vi "fetch frame gige.vi"() -> ()   [LabVIEW 2015]
uses:
  <vilib>/Utility/miscctls.llb/LV3DPointTypeDef.ctl
  <vilib>/Utility/miscctls.llb/LVRGBAColorTypeDef.ctl
  <vilib>/picture/3D Picture Control/Object/Create Object (name).vi
  <userlib>/Mv3dRgbd/Mv3dRgbd.lvlib
  <vilib>/picture/3D Picture Control/NI_3D Picture Control.lvlib
  <userlib>/Mv3dRgbdEx/Mv3dRgbdEx.lvlib
panel:
  in  "value 3":sgl[](array[numeric])
  out "size 5":i32
  out "address 4":i64
  in  "handle":u32
  out "pstU3DeviceInfo out":T1
  out "MV3D_RGBD_GigEDEVICE_INFO out 3":T2(array[cluster])
  out "function return":i32
  out "get list return":i32
  out "pDeviceCount out 2":u32
  out "value 2":u32
  out "open gige function":i32
  out "pstGigeDeviceInfo out 2":T3
  out "MV3D_RGBD_GigEDEVICE_INFO out 2":T4(array[cluster])
  out "get list return 2":i32
  out "pDeviceCount out 3":u32
  out "size 3":i32
  out "address 3":i64
  out "pYuvImgge out":T5
  out "yuv422torgb return":i32
  out "address 2":i64
  out "size 4":i32
  out "address 5":i64
  in  "value":u32
  in  "?":enum32{"RGBD", "点云"}(tab)
  out "RGB":picture
  out "Depth":i16[][](graph)
  out "?":refnum<vi>(3d-picture)
  out "depthtocloud return":i32
  out "handle out 2":u32
  out "pstDepthImage out":T5
  out "fetchframe handle out":u32
  out "fetchframe function":i32
  in  "?":bool
  out "close handle out":u32
  out "close function":i32
  out "start handle out":u32
  out "stop handle out":u32
  out "init function":i32
  out "release function":i32
  out "stop function":i32
  out "start function":i32
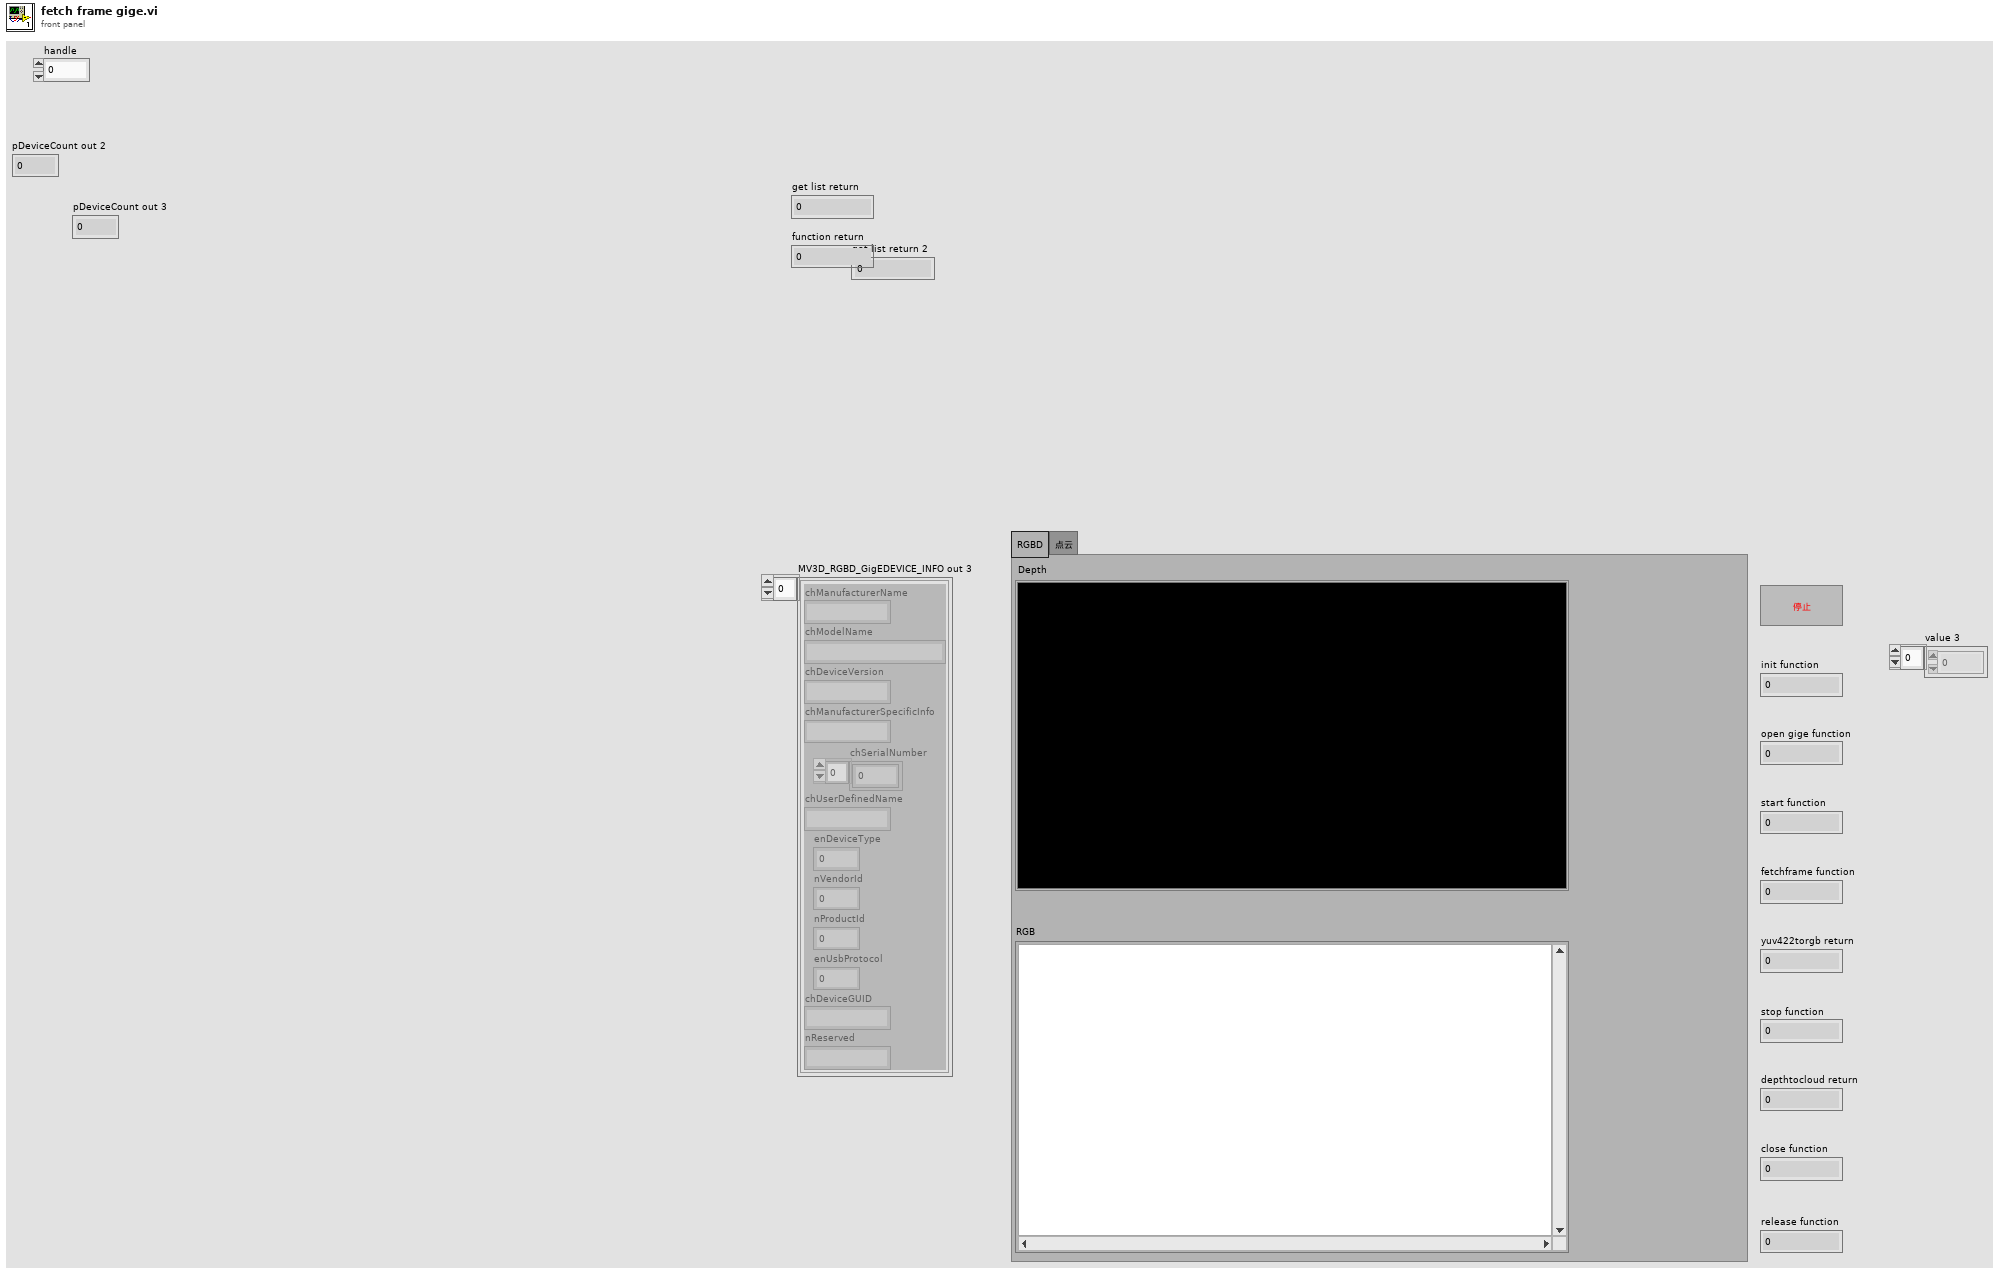
[diagram p1: front panel]
types:
  T1 = cluster{"chManufacturerName[0]":i8, "chManufacturerName[1]":i8, "chManufacturerName[2]":i8, "chManufacturerName[3]":i8, "chManufacturerName[4]":i8, "chManufacturerName[5]":i8, "chManufacturerName[6]":i8, "chManufacturerName[7]":i8, "chManufacturerName[8]":i8, "chManufacturerName[9]":i8, "chManufacturerName[10]":i8, "chManufacturerName[11]":i8, "chManufacturerName[12]":i8, "chManufacturerName[13]":i8, "chManufacturerName[14]":i8, "chManufacturerName[15]":i8, "chManufacturerName[16]":i8, "chManufacturerName[17]":i8, "chManufacturerName[18]":i8, "chManufacturerName[19]":i8, "chManufacturerName[20]":i8, "chManufacturerName[21]":i8, "chManufacturerName[22]":i8, "chManufacturerName[23]":i8, "chManufacturerName[24]":i8, "chManufacturerName[25]":i8, "chManufacturerName[26]":i8, "chManufacturerName[27]":i8, "chManufacturerName[28]":i8, "chManufacturerName[29]":i8, "chManufacturerName[30]":i8, "chManufacturerName[31]":i8, "chModelName[0]":i8, "chModelName[1]":i8, "chModelName[2]":i8, "chModelName[3]":i8, "chModelName[4]":i8, "chModelName[5]":i8, "chModelName[6]":i8, "chModelName[7]":i8, "chModelName[8]":i8, "chModelName[9]":i8, "chModelName[10]":i8, "chModelName[11]":i8, "chModelName[12]":i8, "chModelName[13]":i8, "chModelName[14]":i8, "chModelName[15]":i8, "chModelName[16]":i8, "chModelName[17]":i8, "chModelName[18]":i8, "chModelName[19]":i8, "chModelName[20]":i8, "chModelName[21]":i8, "chModelName[22]":i8, "chModelName[23]":i8, "chModelName[24]":i8, "chModelName[25]":i8, "chModelName[26]":i8, "chModelName[27]":i8, "chModelName[28]":i8, "chModelName[29]":i8, "chModelName[30]":i8, "chModelName[31]":i8, "chDeviceVersion[0]":i8, "chDeviceVersion[1]":i8, "chDeviceVersion[2]":i8, "chDeviceVersion[3]":i8, "chDeviceVersion[4]":i8, "chDeviceVersion[5]":i8, "chDeviceVersion[6]":i8, "chDeviceVersion[7]":i8, "chDeviceVersion[8]":i8, "chDeviceVersion[9]":i8, "chDeviceVersion[10]":i8, "chDeviceVersion[11]":i8, "chDeviceVersion[12]":i8, "chDeviceVersion[13]":i8, "chDeviceVersion[14]":i8, "chDeviceVersion[15]":i8, "chDeviceVersion[16]":i8, "chDeviceVersion[17]":i8, "chDeviceVersion[18]":i8, "chDeviceVersion[19]":i8, "chDeviceVersion[20]":i8, "chDeviceVersion[21]":i8, "chDeviceVersion[22]":i8, "chDeviceVersion[23]":i8, "chDeviceVersion[24]":i8, "chDeviceVersion[25]":i8, "chDeviceVersion[26]":i8, "chDeviceVersion[27]":i8, "chDeviceVersion[28]":i8, "chDeviceVersion[29]":i8, "chDeviceVersion[30]":i8, "chDeviceVersion[31]":i8, "chManufacturerSpecificInfo[0]":i8, "chManufacturerSpecificInfo[1]":i8, "chManufacturerSpecificInfo[2]":i8, "chManufacturerSpecificInfo[3]":i8, "chManufacturerSpecificInfo[4]":i8, "chManufacturerSpecificInfo[5]":i8, "chManufacturerSpecificInfo[6]":i8, "chManufacturerSpecificInfo[7]":i8, "chManufacturerSpecificInfo[8]":i8, "chManufacturerSpecificInfo[9]":i8, "chManufacturerSpecificInfo[10]":i8, "chManufacturerSpecificInfo[11]":i8, "chManufacturerSpecificInfo[12]":i8, "chManufacturerSpecificInfo[13]":i8, "chManufacturerSpecificInfo[14]":i8, "chManufacturerSpecificInfo[15]":i8, "chManufacturerSpecificInfo[16]":i8, "chManufacturerSpecificInfo[17]":i8, "chManufacturerSpecificInfo[18]":i8, "chManufacturerSpecificInfo[19]":i8, "chManufacturerSpecificInfo[20]":i8, "chManufacturerSpecificInfo[21]":i8, "chManufacturerSpecificInfo[22]":i8, "chManufacturerSpecificInfo[23]":i8, "chManufacturerSpecificInfo[24]":i8, "chManufacturerSpecificInfo[25]":i8, "chManufacturerSpecificInfo[26]":i8, "chManufacturerSpecificInfo[27]":i8, "chManufacturerSpecificInfo[28]":i8, "chManufacturerSpecificInfo[29]":i8, "chManufacturerSpecificInfo[30]":i8, "chManufacturerSpecificInfo[31]":i8, "chManufacturerSpecificInfo[32]":i8, "chManufacturerSpecificInfo[33]":i8, "chManufacturerSpecificInfo[34]":i8, "chManufacturerSpecificInfo[35]":i8, "chManufacturerSpecificInfo[36]":i8, "chManufacturerSpecificInfo[37]":i8, "chManufacturerSpecificInfo[38]":i8, "chManufacturerSpecificInfo[39]":i8, "chManufacturerSpecificInfo[40]":i8, "chManufacturerSpecificInfo[41]":i8, "chManufacturerSpecificInfo[42]":i8, "chManufacturerSpecificInfo[43]":i8, "chManufacturerSpecificInfo[44]":i8, "chManufacturerSpecificInfo[45]":i8, "chManufacturerSpecificInfo[46]":i8, "chManufacturerSpecificInfo[47]":i8, "chSerialNumber[0]":i8, "chSerialNumber[1]":i8, "chSerialNumber[2]":i8, "chSerialNumber[3]":i8, "chSerialNumber[4]":i8, "chSerialNumber[5]":i8, "chSerialNumber[6]":i8, "chSerialNumber[7]":i8, "chSerialNumber[8]":i8, "chSerialNumber[9]":i8, "chSerialNumber[10]":i8, "chSerialNumber[11]":i8, "chSerialNumber[12]":i8, "chSerialNumber[13]":i8, "chSerialNumber[14]":i8, "chSerialNumber[15]":i8, "chUserDefinedName[0]":i8, "chUserDefinedName[1]":i8, "chUserDefinedName[2]":i8, "chUserDefinedName[3]":i8, "chUserDefinedName[4]":i8, "chUserDefinedName[5]":i8, "chUserDefinedName[6]":i8, "chUserDefinedName[7]":i8, "chUserDefinedName[8]":i8, "chUserDefinedName[9]":i8, "chUserDefinedName[10]":i8, "chUserDefinedName[11]":i8, "chUserDefinedName[12]":i8, "chUserDefinedName[13]":i8, "chUserDefinedName[14]":i8, "chUserDefinedName[15]":i8, "enDeviceType":i32, "nVendorId":u32, "nProductId":u32, "enUsbProtocol":i32, "chDeviceGUID[0]":i8, "chDeviceGUID[1]":i8, "chDeviceGUID[2]":i8, "chDeviceGUID[3]":i8, "chDeviceGUID[4]":i8, "chDeviceGUID[5]":i8, "chDeviceGUID[6]":i8, "chDeviceGUID[7]":i8, "chDeviceGUID[8]":i8, "chDeviceGUID[9]":i8, "chDeviceGUID[10]":i8, "chDeviceGUID[11]":i8, "chDeviceGUID[12]":i8, "chDeviceGUID[13]":i8, "chDeviceGUID[14]":i8, "chDeviceGUID[15]":i8, "chDeviceGUID[16]":i8, "chDeviceGUID[17]":i8, "chDeviceGUID[18]":i8, "chDeviceGUID[19]":i8, "chDeviceGUID[20]":i8, "chDeviceGUID[21]":i8, "chDeviceGUID[22]":i8, "chDeviceGUID[23]":i8, "chDeviceGUID[24]":i8, "chDeviceGUID[25]":i8, "chDeviceGUID[26]":i8, "chDeviceGUID[27]":i8, "chDeviceGUID[28]":i8, "chDeviceGUID[29]":i8, "chDeviceGUID[30]":i8, "chDeviceGUID[31]":i8, "chDeviceGUID[32]":i8, "chDeviceGUID[33]":i8, "chDeviceGUID[34]":i8, "chDeviceGUID[35]":i8, "chDeviceGUID[36]":i8, "chDeviceGUID[37]":i8, "chDeviceGUID[38]":i8, "chDeviceGUID[39]":i8, "chDeviceGUID[40]":i8, "chDeviceGUID[41]":i8, "chDeviceGUID[42]":i8, "chDeviceGUID[43]":i8, "chDeviceGUID[44]":i8, "chDeviceGUID[45]":i8, "chDeviceGUID[46]":i8, "chDeviceGUID[47]":i8, "chDeviceGUID[48]":i8, "chDeviceGUID[49]":i8, "chDeviceGUID[50]":i8, "chDeviceGUID[51]":i8, "chDeviceGUID[52]":i8, "chDeviceGUID[53]":i8, "chDeviceGUID[54]":i8, "chDeviceGUID[55]":i8, "chDeviceGUID[56]":i8, "chDeviceGUID[57]":i8, "chDeviceGUID[58]":i8, "chDeviceGUID[59]":i8, "chDeviceGUID[60]":i8, "chDeviceGUID[61]":i8, "chDeviceGUID[62]":i8, "chDeviceGUID[63]":i8, "nReserved[0]":u8, "nReserved[1]":u8, "nReserved[2]":u8, "nReserved[3]":u8, "nReserved[4]":u8, "nReserved[5]":u8, "nReserved[6]":u8, "nReserved[7]":u8, "nReserved[8]":u8, "nReserved[9]":u8, "nReserved[10]":u8, "nReserved[11]":u8, "nReserved[12]":u8, "nReserved[13]":u8, "nReserved[14]":u8, "nReserved[15]":u8}
  T2 = cluster{"chManufacturerName":string, "chModelName":string, "chDeviceVersion":string, "chManufacturerSpecificInfo":string, "chSerialNumber":u8[], "chUserDefinedName":string, "enDeviceType":i32, "nVendorId":u32, "nProductId":u32, "enUsbProtocol":i32, "chDeviceGUID":string, "nReserved":string}[]
  T3 = cluster{"chManufacturerName[0]":i8, "chManufacturerName[1]":i8, "chManufacturerName[2]":i8, "chManufacturerName[3]":i8, "chManufacturerName[4]":i8, "chManufacturerName[5]":i8, "chManufacturerName[6]":i8, "chManufacturerName[7]":i8, "chManufacturerName[8]":i8, "chManufacturerName[9]":i8, "chManufacturerName[10]":i8, "chManufacturerName[11]":i8, "chManufacturerName[12]":i8, "chManufacturerName[13]":i8, "chManufacturerName[14]":i8, "chManufacturerName[15]":i8, "chManufacturerName[16]":i8, "chManufacturerName[17]":i8, "chManufacturerName[18]":i8, "chManufacturerName[19]":i8, "chManufacturerName[20]":i8, "chManufacturerName[21]":i8, "chManufacturerName[22]":i8, "chManufacturerName[23]":i8, "chManufacturerName[24]":i8, "chManufacturerName[25]":i8, "chManufacturerName[26]":i8, "chManufacturerName[27]":i8, "chManufacturerName[28]":i8, "chManufacturerName[29]":i8, "chManufacturerName[30]":i8, "chManufacturerName[31]":i8, "chModelName[0]":i8, "chModelName[1]":i8, "chModelName[2]":i8, "chModelName[3]":i8, "chModelName[4]":i8, "chModelName[5]":i8, "chModelName[6]":i8, "chModelName[7]":i8, "chModelName[8]":i8, "chModelName[9]":i8, "chModelName[10]":i8, "chModelName[11]":i8, "chModelName[12]":i8, "chModelName[13]":i8, "chModelName[14]":i8, "chModelName[15]":i8, "chModelName[16]":i8, "chModelName[17]":i8, "chModelName[18]":i8, "chModelName[19]":i8, "chModelName[20]":i8, "chModelName[21]":i8, "chModelName[22]":i8, "chModelName[23]":i8, "chModelName[24]":i8, "chModelName[25]":i8, "chModelName[26]":i8, "chModelName[27]":i8, "chModelName[28]":i8, "chModelName[29]":i8, "chModelName[30]":i8, "chModelName[31]":i8, "chDeviceVersion[0]":i8, "chDeviceVersion[1]":i8, "chDeviceVersion[2]":i8, "chDeviceVersion[3]":i8, "chDeviceVersion[4]":i8, "chDeviceVersion[5]":i8, "chDeviceVersion[6]":i8, "chDeviceVersion[7]":i8, "chDeviceVersion[8]":i8, "chDeviceVersion[9]":i8, "chDeviceVersion[10]":i8, "chDeviceVersion[11]":i8, "chDeviceVersion[12]":i8, "chDeviceVersion[13]":i8, "chDeviceVersion[14]":i8, "chDeviceVersion[15]":i8, "chDeviceVersion[16]":i8, "chDeviceVersion[17]":i8, "chDeviceVersion[18]":i8, "chDeviceVersion[19]":i8, "chDeviceVersion[20]":i8, "chDeviceVersion[21]":i8, "chDeviceVersion[22]":i8, "chDeviceVersion[23]":i8, "chDeviceVersion[24]":i8, "chDeviceVersion[25]":i8, "chDeviceVersion[26]":i8, "chDeviceVersion[27]":i8, "chDeviceVersion[28]":i8, "chDeviceVersion[29]":i8, "chDeviceVersion[30]":i8, "chDeviceVersion[31]":i8, "chManufacturerSpecificInfo[0]":i8, "chManufacturerSpecificInfo[1]":i8, "chManufacturerSpecificInfo[2]":i8, "chManufacturerSpecificInfo[3]":i8, "chManufacturerSpecificInfo[4]":i8, "chManufacturerSpecificInfo[5]":i8, "chManufacturerSpecificInfo[6]":i8, "chManufacturerSpecificInfo[7]":i8, "chManufacturerSpecificInfo[8]":i8, "chManufacturerSpecificInfo[9]":i8, "chManufacturerSpecificInfo[10]":i8, "chManufacturerSpecificInfo[11]":i8, "chManufacturerSpecificInfo[12]":i8, "chManufacturerSpecificInfo[13]":i8, "chManufacturerSpecificInfo[14]":i8, "chManufacturerSpecificInfo[15]":i8, "chManufacturerSpecificInfo[16]":i8, "chManufacturerSpecificInfo[17]":i8, "chManufacturerSpecificInfo[18]":i8, "chManufacturerSpecificInfo[19]":i8, "chManufacturerSpecificInfo[20]":i8, "chManufacturerSpecificInfo[21]":i8, "chManufacturerSpecificInfo[22]":i8, "chManufacturerSpecificInfo[23]":i8, "chManufacturerSpecificInfo[24]":i8, "chManufacturerSpecificInfo[25]":i8, "chManufacturerSpecificInfo[26]":i8, "chManufacturerSpecificInfo[27]":i8, "chManufacturerSpecificInfo[28]":i8, "chManufacturerSpecificInfo[29]":i8, "chManufacturerSpecificInfo[30]":i8, "chManufacturerSpecificInfo[31]":i8, "chManufacturerSpecificInfo[32]":i8, "chManufacturerSpecificInfo[33]":i8, "chManufacturerSpecificInfo[34]":i8, "chManufacturerSpecificInfo[35]":i8, "chManufacturerSpecificInfo[36]":i8, "chManufacturerSpecificInfo[37]":i8, "chManufacturerSpecificInfo[38]":i8, "chManufacturerSpecificInfo[39]":i8, "chManufacturerSpecificInfo[40]":i8, "chManufacturerSpecificInfo[41]":i8, "chManufacturerSpecificInfo[42]":i8, "chManufacturerSpecificInfo[43]":i8, "chManufacturerSpecificInfo[44]":i8, "chManufacturerSpecificInfo[45]":i8, "chManufacturerSpecificInfo[46]":i8, "chManufacturerSpecificInfo[47]":i8, "chSerialNumber[0]":i8, "chSerialNumber[1]":i8, "chSerialNumber[2]":i8, "chSerialNumber[3]":i8, "chSerialNumber[4]":i8, "chSerialNumber[5]":i8, "chSerialNumber[6]":i8, "chSerialNumber[7]":i8, "chSerialNumber[8]":i8, "chSerialNumber[9]":i8, "chSerialNumber[10]":i8, "chSerialNumber[11]":i8, "chSerialNumber[12]":i8, "chSerialNumber[13]":i8, "chSerialNumber[14]":i8, "chSerialNumber[15]":i8, "chUserDefinedName[0]":i8, "chUserDefinedName[1]":i8, "chUserDefinedName[2]":i8, "chUserDefinedName[3]":i8, "chUserDefinedName[4]":i8, "chUserDefinedName[5]":i8, "chUserDefinedName[6]":i8, "chUserDefinedName[7]":i8, "chUserDefinedName[8]":i8, "chUserDefinedName[9]":i8, "chUserDefinedName[10]":i8, "chUserDefinedName[11]":i8, "chUserDefinedName[12]":i8, "chUserDefinedName[13]":i8, "chUserDefinedName[14]":i8, "chUserDefinedName[15]":i8, "enDeviceType":i32, "chMacAddress[0]":u8, "chMacAddress[1]":u8, "chMacAddress[2]":u8, "chMacAddress[3]":u8, "chMacAddress[4]":u8, "chMacAddress[5]":u8, "chMacAddress[6]":u8, "chMacAddress[7]":u8, "enIPCfgMode":i32, "chCurrentIp[0]":i8, "chCurrentIp[1]":i8, "chCurrentIp[2]":i8, "chCurrentIp[3]":i8, "chCurrentIp[4]":i8, "chCurrentIp[5]":i8, "chCurrentIp[6]":i8, "chCurrentIp[7]":i8, "chCurrentIp[8]":i8, "chCurrentIp[9]":i8, "chCurrentIp[10]":i8, "chCurrentIp[11]":i8, "chCurrentIp[12]":i8, "chCurrentIp[13]":i8, "chCurrentIp[14]":i8, "chCurrentIp[15]":i8, "chCurrentSubNetMask[0]":i8, "chCurrentSubNetMask[1]":i8, "chCurrentSubNetMask[2]":i8, "chCurrentSubNetMask[3]":i8, "chCurrentSubNetMask[4]":i8, "chCurrentSubNetMask[5]":i8, "chCurrentSubNetMask[6]":i8, "chCurrentSubNetMask[7]":i8, "chCurrentSubNetMask[8]":i8, "chCurrentSubNetMask[9]":i8, "chCurrentSubNetMask[10]":i8, "chCurrentSubNetMask[11]":i8, "chCurrentSubNetMask[12]":i8, "chCurrentSubNetMask[13]":i8, "chCurrentSubNetMask[14]":i8, "chCurrentSubNetMask[15]":i8, "chDefultGateWay[0]":i8, "chDefultGateWay[1]":i8, "chDefultGateWay[2]":i8, "chDefultGateWay[3]":i8, "chDefultGateWay[4]":i8, "chDefultGateWay[5]":i8, "chDefultGateWay[6]":i8, "chDefultGateWay[7]":i8, "chDefultGateWay[8]":i8, "chDefultGateWay[9]":i8, "chDefultGateWay[10]":i8, "chDefultGateWay[11]":i8, "chDefultGateWay[12]":i8, "chDefultGateWay[13]":i8, "chDefultGateWay[14]":i8, "chDefultGateWay[15]":i8, "chNetExport[0]":i8, "chNetExport[1]":i8, "chNetExport[2]":i8, "chNetExport[3]":i8, "chNetExport[4]":i8, "chNetExport[5]":i8, "chNetExport[6]":i8, "chNetExport[7]":i8, "chNetExport[8]":i8, "chNetExport[9]":i8, "chNetExport[10]":i8, "chNetExport[11]":i8, "chNetExport[12]":i8, "chNetExport[13]":i8, "chNetExport[14]":i8, "chNetExport[15]":i8, "nReserved[0]":u8, "nReserved[1]":u8, "nReserved[2]":u8, "nReserved[3]":u8, "nReserved[4]":u8, "nReserved[5]":u8, "nReserved[6]":u8, "nReserved[7]":u8, "nReserved[8]":u8, "nReserved[9]":u8, "nReserved[10]":u8, "nReserved[11]":u8, "nReserved[12]":u8, "nReserved[13]":u8, "nReserved[14]":u8, "nReserved[15]":u8}
  T4 = cluster{"chManufacturerName":string, "chModelName":string, "chDeviceVersion":string, "chManufacturerSpecificInfo":string, "chSerialNumber":u8[], "chUserDefinedName":string, "enDeviceType":i32, "chMacAddress":u8[], "enIPCfgMode":i32, "chCurrentIp":string, "chCurrentSubNetMask":string, "chDefultGateWay":string, "chNetExport":string, "nReserved":string}[]
  T5 = cluster{"enImageType":i32, "nWidth":u32, "nHeight":u32, "pData":u32, "nDataLen":u32, "nFrameNum":u32, "nTimeStamp":i64, "nReserved[0]":u8, "nReserved[1]":u8, "nReserved[2]":u8, "nReserved[3]":u8, "nReserved[4]":u8, "nReserved[5]":u8, "nReserved[6]":u8, "nReserved[7]":u8, "nReserved[8]":u8, "nReserved[9]":u8, "nReserved[10]":u8, "nReserved[11]":u8, "nReserved[12]":u8, "nReserved[13]":u8, "nReserved[14]":u8, "nReserved[15]":u8}
  T6 = typedef "LVRGBAColorTypeDef.ctl" = cluster{"Red":sgl, "Green":sgl, "Blue":sgl, "Alpha":sgl}
  T7 = typedef "LV3DPointTypeDef.ctl" = cluster{"X":sgl, "Y":sgl, "Z":sgl}
  T8 = cluster{"nImageCount":u64, "MV3D_RGBD_IMAGE_DATA[0]":cluster{"enImageType":i32, "nWidth":u32, "nHeight":u32, "pData":u32, "nDataLen":u32, "nFrameNum":u32, "nTimeStamp":i64, "nReserved[0]":u8, "nReserved[1]":u8, "nReserved[2]":u8, "nReserved[3]":u8, "nReserved[4]":u8, "nReserved[5]":u8, "nReserved[6]":u8, "nReserved[7]":u8, "nReserved[8]":u8, "nReserved[9]":u8, "nReserved[10]":u8, "nReserved[11]":u8, "nReserved[12]":u8, "nReserved[13]":u8, "nReserved[14]":u8, "nReserved[15]":u8}, "MV3D_RGBD_IMAGE_DATA[1]":cluster{"enImageType":i32, "nWidth":u32, "nHeight":u32, "pData":u32, "nDataLen":u32, "nFrameNum":u32, "nTimeStamp":i64, "nReserved[0]":u8, "nReserved[1]":u8, "nReserved[2]":u8, "nReserved[3]":u8, "nReserved[4]":u8, "nReserved[5]":u8, "nReserved[6]":u8, "nReserved[7]":u8, "nReserved[8]":u8, "nReserved[9]":u8, "nReserved[10]":u8, "nReserved[11]":u8, "nReserved[12]":u8, "nReserved[13]":u8, "nReserved[14]":u8, "nReserved[15]":u8}, "MV3D_RGBD_IMAGE_DATA[2]":cluster{"enImageType":i32, "nWidth":u32, "nHeight":u32, "pData":u32, "nDataLen":u32, "nFrameNum":u32, "nTimeStamp":i64, "nReserved[0]":u8, "nReserved[1]":u8, "nReserved[2]":u8, "nReserved[3]":u8, "nReserved[4]":u8, "nReserved[5]":u8, "nReserved[6]":u8, "nReserved[7]":u8, "nReserved[8]":u8, "nReserved[9]":u8, "nReserved[10]":u8, "nReserved[11]":u8, "nReserved[12]":u8, "nReserved[13]":u8, "nReserved[14]":u8, "nReserved[15]":u8}, "MV3D_RGBD_IMAGE_DATA[3]":cluster{"enImageType":i32, "nWidth":u32, "nHeight":u32, "pData":u32, "nDataLen":u32, "nFrameNum":u32, "nTimeStamp":i64, "nReserved[0]":u8, "nReserved[1]":u8, "nReserved[2]":u8, "nReserved[3]":u8, "nReserved[4]":u8, "nReserved[5]":u8, "nReserved[6]":u8, "nReserved[7]":u8, "nReserved[8]":u8, "nReserved[9]":u8, "nReserved[10]":u8, "nReserved[11]":u8, "nReserved[12]":u8, "nReserved[13]":u8, "nReserved[14]":u8, "nReserved[15]":u8}, "MV3D_RGBD_IMAGE_DATA[4]":cluster{"enImageType":i32, "nWidth":u32, "nHeight":u32, "pData":u32, "nDataLen":u32, "nFrameNum":u32, "nTimeStamp":i64, "nReserved[0]":u8, "nReserved[1]":u8, "nReserved[2]":u8, "nReserved[3]":u8, "nReserved[4]":u8, "nReserved[5]":u8, "nReserved[6]":u8, "nReserved[7]":u8, "nReserved[8]":u8, "nReserved[9]":u8, "nReserved[10]":u8, "nReserved[11]":u8, "nReserved[12]":u8, "nReserved[13]":u8, "nReserved[14]":u8, "nReserved[15]":u8}, "MV3D_RGBD_IMAGE_DATA[5]":cluster{"enImageType":i32, "nWidth":u32, "nHeight":u32, "pData":u32, "nDataLen":u32, "nFrameNum":u32, "nTimeStamp":i64, "nReserved[0]":u8, "nReserved[1]":u8, "nReserved[2]":u8, "nReserved[3]":u8, "nReserved[4]":u8, "nReserved[5]":u8, "nReserved[6]":u8, "nReserved[7]":u8, "nReserved[8]":u8, "nReserved[9]":u8, "nReserved[10]":u8, "nReserved[11]":u8, "nReserved[12]":u8, "nReserved[13]":u8, "nReserved[14]":u8, "nReserved[15]":u8}, "MV3D_RGBD_IMAGE_DATA[6]":cluster{"enImageType":i32, "nWidth":u32, "nHeight":u32, "pData":u32, "nDataLen":u32, "nFrameNum":u32, "nTimeStamp":i64, "nReserved[0]":u8, "nReserved[1]":u8, "nReserved[2]":u8, "nReserved[3]":u8, "nReserved[4]":u8, "nReserved[5]":u8, "nReserved[6]":u8, "nReserved[7]":u8, "nReserved[8]":u8, "nReserved[9]":u8, "nReserved[10]":u8, "nReserved[11]":u8, "nReserved[12]":u8, "nReserved[13]":u8, "nReserved[14]":u8, "nReserved[15]":u8}, "MV3D_RGBD_IMAGE_DATA[7]":cluster{"enImageType":i32, "nWidth":u32, "nHeight":u32, "pData":u32, "nDataLen":u32, "nFrameNum":u32, "nTimeStamp":i64, "nReserved[0]":u8, "nReserved[1]":u8, "nReserved[2]":u8, "nReserved[3]":u8, "nReserved[4]":u8, "nReserved[5]":u8, "nReserved[6]":u8, "nReserved[7]":u8, "nReserved[8]":u8, "nReserved[9]":u8, "nReserved[10]":u8, "nReserved[11]":u8, "nReserved[12]":u8, "nReserved[13]":u8, "nReserved[14]":u8, "nReserved[15]":u8}, "MV3D_RGBD_IMAGE_DATA[8]":cluster{"enImageType":i32, "nWidth":u32, "nHeight":u32, "pData":u32, "nDataLen":u32, "nFrameNum":u32, "nTimeStamp":i64, "nReserved[0]":u8, "nReserved[1]":u8, "nReserved[2]":u8, "nReserved[3]":u8, "nReserved[4]":u8, "nReserved[5]":u8, "nReserved[6]":u8, "nReserved[7]":u8, "nReserved[8]":u8, "nReserved[9]":u8, "nReserved[10]":u8, "nReserved[11]":u8, "nReserved[12]":u8, "nReserved[13]":u8, "nReserved[14]":u8, "nReserved[15]":u8}, "MV3D_RGBD_IMAGE_DATA[9]":cluster{"enImageType":i32, "nWidth":u32, "nHeight":u32, "pData":u32, "nDataLen":u32, "nFrameNum":u32, "nTimeStamp":i64, "nReserved[0]":u8, "nReserved[1]":u8, "nReserved[2]":u8, "nReserved[3]":u8, "nReserved[4]":u8, "nReserved[5]":u8, "nReserved[6]":u8, "nReserved[7]":u8, "nReserved[8]":u8, "nReserved[9]":u8, "nReserved[10]":u8, "nReserved[11]":u8, "nReserved[12]":u8, "nReserved[13]":u8, "nReserved[14]":u8, "nReserved[15]":u8}, "nReserved[0]":u8, "nReserved[1]":u8, "nReserved[2]":u8, "nReserved[3]":u8, "nReserved[4]":u8, "nReserved[5]":u8, "nReserved[6]":u8, "nReserved[7]":u8, "nReserved[8]":u8, "nReserved[9]":u8, "nReserved[10]":u8, "nReserved[11]":u8, "nReserved[12]":u8, "nReserved[13]":u8, "nReserved[14]":u8, "nReserved[15]":u8}
  T9 = enum16{"Overall", "Per Primitive", "Per Vertex", "Binding Off"}
  T10 = enum16{"Points", "Lines", "Line Strip", "Line Loop", "Triangles", "Triangle Strip", "Triangle Fan", "Quads", "Quad Strip", "Polygon"}
  T11 = cluster{"chManufacturerName[0]":i8, "chManufacturerName[1]":i8, "chManufacturerName[2]":i8, "chManufacturerName[3]":i8, "chManufacturerName[4]":i8, "chManufacturerName[5]":i8, "chManufacturerName[6]":i8, "chManufacturerName[7]":i8, "chManufacturerName[8]":i8, "chManufacturerName[9]":i8, "chManufacturerName[10]":i8, "chManufacturerName[11]":i8, "chManufacturerName[12]":i8, "chManufacturerName[13]":i8, "chManufacturerName[14]":i8, "chManufacturerName[15]":i8, "chManufacturerName[16]":i8, "chManufacturerName[17]":i8, "chManufacturerName[18]":i8, "chManufacturerName[19]":i8, "chManufacturerName[20]":i8, "chManufacturerName[21]":i8, "chManufacturerName[22]":i8, "chManufacturerName[23]":i8, "chManufacturerName[24]":i8, "chManufacturerName[25]":i8, "chManufacturerName[26]":i8, "chManufacturerName[27]":i8, "chManufacturerName[28]":i8, "chManufacturerName[29]":i8, "chManufacturerName[30]":i8, "chManufacturerName[31]":i8, "chModelName[0]":i8, "chModelName[1]":i8, "chModelName[2]":i8, "chModelName[3]":i8, "chModelName[4]":i8, "chModelName[5]":i8, "chModelName[6]":i8, "chModelName[7]":i8, "chModelName[8]":i8, "chModelName[9]":i8, "chModelName[10]":i8, "chModelName[11]":i8, "chModelName[12]":i8, "chModelName[13]":i8, "chModelName[14]":i8, "chModelName[15]":i8, "chModelName[16]":i8, "chModelName[17]":i8, "chModelName[18]":i8, "chModelName[19]":i8, "chModelName[20]":i8, "chModelName[21]":i8, "chModelName[22]":i8, "chModelName[23]":i8, "chModelName[24]":i8, "chModelName[25]":i8, "chModelName[26]":i8, "chModelName[27]":i8, "chModelName[28]":i8, "chModelName[29]":i8, "chModelName[30]":i8, "chModelName[31]":i8, "chDeviceVersion[0]":i8, "chDeviceVersion[1]":i8, "chDeviceVersion[2]":i8, "chDeviceVersion[3]":i8, "chDeviceVersion[4]":i8, "chDeviceVersion[5]":i8, "chDeviceVersion[6]":i8, "chDeviceVersion[7]":i8, "chDeviceVersion[8]":i8, "chDeviceVersion[9]":i8, "chDeviceVersion[10]":i8, "chDeviceVersion[11]":i8, "chDeviceVersion[12]":i8, "chDeviceVersion[13]":i8, "chDeviceVersion[14]":i8, "chDeviceVersion[15]":i8, "chDeviceVersion[16]":i8, "chDeviceVersion[17]":i8, "chDeviceVersion[18]":i8, "chDeviceVersion[19]":i8, "chDeviceVersion[20]":i8, "chDeviceVersion[21]":i8, "chDeviceVersion[22]":i8, "chDeviceVersion[23]":i8, "chDeviceVersion[24]":i8, "chDeviceVersion[25]":i8, "chDeviceVersion[26]":i8, "chDeviceVersion[27]":i8, "chDeviceVersion[28]":i8, "chDeviceVersion[29]":i8, "chDeviceVersion[30]":i8, "chDeviceVersion[31]":i8, "chManufacturerSpecificInfo[0]":i8, "chManufacturerSpecificInfo[1]":i8, "chManufacturerSpecificInfo[2]":i8, "chManufacturerSpecificInfo[3]":i8, "chManufacturerSpecificInfo[4]":i8, "chManufacturerSpecificInfo[5]":i8, "chManufacturerSpecificInfo[6]":i8, "chManufacturerSpecificInfo[7]":i8, "chManufacturerSpecificInfo[8]":i8, "chManufacturerSpecificInfo[9]":i8, "chManufacturerSpecificInfo[10]":i8, "chManufacturerSpecificInfo[11]":i8, "chManufacturerSpecificInfo[12]":i8, "chManufacturerSpecificInfo[13]":i8, "chManufacturerSpecificInfo[14]":i8, "chManufacturerSpecificInfo[15]":i8, "chManufacturerSpecificInfo[16]":i8, "chManufacturerSpecificInfo[17]":i8, "chManufacturerSpecificInfo[18]":i8, "chManufacturerSpecificInfo[19]":i8, "chManufacturerSpecificInfo[20]":i8, "chManufacturerSpecificInfo[21]":i8, "chManufacturerSpecificInfo[22]":i8, "chManufacturerSpecificInfo[23]":i8, "chManufacturerSpecificInfo[24]":i8, "chManufacturerSpecificInfo[25]":i8, "chManufacturerSpecificInfo[26]":i8, "chManufacturerSpecificInfo[27]":i8, "chManufacturerSpecificInfo[28]":i8, "chManufacturerSpecificInfo[29]":i8, "chManufacturerSpecificInfo[30]":i8, "chManufacturerSpecificInfo[31]":i8, "chManufacturerSpecificInfo[32]":i8, "chManufacturerSpecificInfo[33]":i8, "chManufacturerSpecificInfo[34]":i8, "chManufacturerSpecificInfo[35]":i8, "chManufacturerSpecificInfo[36]":i8, "chManufacturerSpecificInfo[37]":i8, "chManufacturerSpecificInfo[38]":i8, "chManufacturerSpecificInfo[39]":i8, "chManufacturerSpecificInfo[40]":i8, "chManufacturerSpecificInfo[41]":i8, "chManufacturerSpecificInfo[42]":i8, "chManufacturerSpecificInfo[43]":i8, "chManufacturerSpecificInfo[44]":i8, "chManufacturerSpecificInfo[45]":i8, "chManufacturerSpecificInfo[46]":i8, "chManufacturerSpecificInfo[47]":i8, "chSerialNumber[0]":i8, "chSerialNumber[1]":i8, "chSerialNumber[2]":i8, "chSerialNumber[3]":i8, "chSerialNumber[4]":i8, "chSerialNumber[5]":i8, "chSerialNumber[6]":i8, "chSerialNumber[7]":i8, "chSerialNumber[8]":i8, "chSerialNumber[9]":i8, "chSerialNumber[10]":i8, "chSerialNumber[11]":i8, "chSerialNumber[12]":i8, "chSerialNumber[13]":i8, "chSerialNumber[14]":i8, "chSerialNumber[15]":i8, "chUserDefinedName[0]":i8, "chUserDefinedName[1]":i8, "chUserDefinedName[2]":i8, "chUserDefinedName[3]":i8, "chUserDefinedName[4]":i8, "chUserDefinedName[5]":i8, "chUserDefinedName[6]":i8, "chUserDefinedName[7]":i8, "chUserDefinedName[8]":i8, "chUserDefinedName[9]":i8, "chUserDefinedName[10]":i8, "chUserDefinedName[11]":i8, "chUserDefinedName[12]":i8, "chUserDefinedName[13]":i8, "chUserDefinedName[14]":i8, "chUserDefinedName[15]":i8, "enDeviceType":i32, "chMacAddress[0]":u8, "chMacAddress[1]":u8, "chMacAddress[2]":u8, "chMacAddress[3]":u8, "chMacAddress[4]":u8, "chMacAddress[5]":u8, "chMacAddress[6]":u8, "chMacAddress[7]":u8, "enIPCfgMode":i32, "chCurrentIp[0]":i8, "chCurrentIp[1]":i8, "chCurrentIp[2]":i8, "chCurrentIp[3]":i8, "chCurrentIp[4]":i8, "chCurrentIp[5]":i8, "chCurrentIp[6]":i8, "chCurrentIp[7]":i8, "chCurrentIp[8]":i8, "chCurrentIp[9]":i8, "chCurrentIp[10]":i8, "chCurrentIp[11]":i8, "chCurrentIp[12]":i8, "chCurrentIp[13]":i8, "chCurrentIp[14]":i8, "chCurrentIp[15]":i8, "chCurrentSubNetMask[0]":i8, "chCurrentSubNetMask[1]":i8, "chCurrentSubNetMask[2]":i8, "chCurrentSubNetMask[3]":i8, "chCurrentSubNetMask[4]":i8, "chCurrentSubNetMask[5]":i8, "chCurrentSubNetMask[6]":i8, "chCurrentSubNetMask[7]":i8, "chCurrentSubNetMask[8]":i8, "chCurrentSubNetMask[9]":i8, "chCurrentSubNetMask[10]":i8, "chCurrentSubNetMask[11]":i8, "chCurrentSubNetMask[12]":i8, "chCurrentSubNetMask[13]":i8, "chCurrentSubNetMask[14]":i8, "chCurrentSubNetMask[15]":i8, "chDefultGateWay[0]":i8, "chDefultGateWay[1]":i8, "chDefultGateWay[2]":i8, "chDefultGateWay[3]":i8, "chDefultGateWay[4]":i8, "chDefultGateWay[5]":i8, "chDefultGateWay[6]":i8, "chDefultGateWay[7]":i8, "chDefultGateWay[8]":i8, "chDefultGateWay[9]":i8, "chDefultGateWay[10]":i8, "chDefultGateWay[11]":i8, "chDefultGateWay[12]":i8, "chDefultGateWay[13]":i8, "chDefultGateWay[14]":i8, "chDefultGateWay[15]":i8, "chNetExport[0]":i8, "chNetExport[1]":i8, "chNetExport[2]":i8, "chNetExport[3]":i8, "chNetExport[4]":i8, "chNetExport[5]":i8, "chNetExport[6]":i8, "chNetExport[7]":i8, "chNetExport[8]":i8, "chNetExport[9]":i8, "chNetExport[10]":i8, "chNetExport[11]":i8, "chNetExport[12]":i8, "chNetExport[13]":i8, "chNetExport[14]":i8, "chNetExport[15]":i8, "nReserved[0]":u8, "nReserved[1]":u8, "nReserved[2]":u8, "nReserved[3]":u8, "nReserved[4]":u8, "nReserved[5]":u8, "nReserved[6]":u8, "nReserved[7]":u8, "nReserved[8]":u8, "nReserved[9]":u8, "nReserved[10]":u8, "nReserved[11]":u8, "nReserved[12]":u8, "nReserved[13]":u8, "nReserved[14]":u8, "nReserved[15]":u8}[]
  T12 = cluster{"chManufacturerName[0]":i8, "chManufacturerName[1]":i8, "chManufacturerName[2]":i8, "chManufacturerName[3]":i8, "chManufacturerName[4]":i8, "chManufacturerName[5]":i8, "chManufacturerName[6]":i8, "chManufacturerName[7]":i8, "chManufacturerName[8]":i8, "chManufacturerName[9]":i8, "chManufacturerName[10]":i8, "chManufacturerName[11]":i8, "chManufacturerName[12]":i8, "chManufacturerName[13]":i8, "chManufacturerName[14]":i8, "chManufacturerName[15]":i8, "chManufacturerName[16]":i8, "chManufacturerName[17]":i8, "chManufacturerName[18]":i8, "chManufacturerName[19]":i8, "chManufacturerName[20]":i8, "chManufacturerName[21]":i8, "chManufacturerName[22]":i8, "chManufacturerName[23]":i8, "chManufacturerName[24]":i8, "chManufacturerName[25]":i8, "chManufacturerName[26]":i8, "chManufacturerName[27]":i8, "chManufacturerName[28]":i8, "chManufacturerName[29]":i8, "chManufacturerName[30]":i8, "chManufacturerName[31]":i8, "chModelName[0]":i8, "chModelName[1]":i8, "chModelName[2]":i8, "chModelName[3]":i8, "chModelName[4]":i8, "chModelName[5]":i8, "chModelName[6]":i8, "chModelName[7]":i8, "chModelName[8]":i8, "chModelName[9]":i8, "chModelName[10]":i8, "chModelName[11]":i8, "chModelName[12]":i8, "chModelName[13]":i8, "chModelName[14]":i8, "chModelName[15]":i8, "chModelName[16]":i8, "chModelName[17]":i8, "chModelName[18]":i8, "chModelName[19]":i8, "chModelName[20]":i8, "chModelName[21]":i8, "chModelName[22]":i8, "chModelName[23]":i8, "chModelName[24]":i8, "chModelName[25]":i8, "chModelName[26]":i8, "chModelName[27]":i8, "chModelName[28]":i8, "chModelName[29]":i8, "chModelName[30]":i8, "chModelName[31]":i8, "chDeviceVersion[0]":i8, "chDeviceVersion[1]":i8, "chDeviceVersion[2]":i8, "chDeviceVersion[3]":i8, "chDeviceVersion[4]":i8, "chDeviceVersion[5]":i8, "chDeviceVersion[6]":i8, "chDeviceVersion[7]":i8, "chDeviceVersion[8]":i8, "chDeviceVersion[9]":i8, "chDeviceVersion[10]":i8, "chDeviceVersion[11]":i8, "chDeviceVersion[12]":i8, "chDeviceVersion[13]":i8, "chDeviceVersion[14]":i8, "chDeviceVersion[15]":i8, "chDeviceVersion[16]":i8, "chDeviceVersion[17]":i8, "chDeviceVersion[18]":i8, "chDeviceVersion[19]":i8, "chDeviceVersion[20]":i8, "chDeviceVersion[21]":i8, "chDeviceVersion[22]":i8, "chDeviceVersion[23]":i8, "chDeviceVersion[24]":i8, "chDeviceVersion[25]":i8, "chDeviceVersion[26]":i8, "chDeviceVersion[27]":i8, "chDeviceVersion[28]":i8, "chDeviceVersion[29]":i8, "chDeviceVersion[30]":i8, "chDeviceVersion[31]":i8, "chManufacturerSpecificInfo[0]":i8, "chManufacturerSpecificInfo[1]":i8, "chManufacturerSpecificInfo[2]":i8, "chManufacturerSpecificInfo[3]":i8, "chManufacturerSpecificInfo[4]":i8, "chManufacturerSpecificInfo[5]":i8, "chManufacturerSpecificInfo[6]":i8, "chManufacturerSpecificInfo[7]":i8, "chManufacturerSpecificInfo[8]":i8, "chManufacturerSpecificInfo[9]":i8, "chManufacturerSpecificInfo[10]":i8, "chManufacturerSpecificInfo[11]":i8, "chManufacturerSpecificInfo[12]":i8, "chManufacturerSpecificInfo[13]":i8, "chManufacturerSpecificInfo[14]":i8, "chManufacturerSpecificInfo[15]":i8, "chManufacturerSpecificInfo[16]":i8, "chManufacturerSpecificInfo[17]":i8, "chManufacturerSpecificInfo[18]":i8, "chManufacturerSpecificInfo[19]":i8, "chManufacturerSpecificInfo[20]":i8, "chManufacturerSpecificInfo[21]":i8, "chManufacturerSpecificInfo[22]":i8, "chManufacturerSpecificInfo[23]":i8, "chManufacturerSpecificInfo[24]":i8, "chManufacturerSpecificInfo[25]":i8, "chManufacturerSpecificInfo[26]":i8, "chManufacturerSpecificInfo[27]":i8, "chManufacturerSpecificInfo[28]":i8, "chManufacturerSpecificInfo[29]":i8, "chManufacturerSpecificInfo[30]":i8, "chManufacturerSpecificInfo[31]":i8, "chManufacturerSpecificInfo[32]":i8, "chManufacturerSpecificInfo[33]":i8, "chManufacturerSpecificInfo[34]":i8, "chManufacturerSpecificInfo[35]":i8, "chManufacturerSpecificInfo[36]":i8, "chManufacturerSpecificInfo[37]":i8, "chManufacturerSpecificInfo[38]":i8, "chManufacturerSpecificInfo[39]":i8, "chManufacturerSpecificInfo[40]":i8, "chManufacturerSpecificInfo[41]":i8, "chManufacturerSpecificInfo[42]":i8, "chManufacturerSpecificInfo[43]":i8, "chManufacturerSpecificInfo[44]":i8, "chManufacturerSpecificInfo[45]":i8, "chManufacturerSpecificInfo[46]":i8, "chManufacturerSpecificInfo[47]":i8, "chSerialNumber[0]":i8, "chSerialNumber[1]":i8, "chSerialNumber[2]":i8, "chSerialNumber[3]":i8, "chSerialNumber[4]":i8, "chSerialNumber[5]":i8, "chSerialNumber[6]":i8, "chSerialNumber[7]":i8, "chSerialNumber[8]":i8, "chSerialNumber[9]":i8, "chSerialNumber[10]":i8, "chSerialNumber[11]":i8, "chSerialNumber[12]":i8, "chSerialNumber[13]":i8, "chSerialNumber[14]":i8, "chSerialNumber[15]":i8, "chUserDefinedName[0]":i8, "chUserDefinedName[1]":i8, "chUserDefinedName[2]":i8, "chUserDefinedName[3]":i8, "chUserDefinedName[4]":i8, "chUserDefinedName[5]":i8, "chUserDefinedName[6]":i8, "chUserDefinedName[7]":i8, "chUserDefinedName[8]":i8, "chUserDefinedName[9]":i8, "chUserDefinedName[10]":i8, "chUserDefinedName[11]":i8, "chUserDefinedName[12]":i8, "chUserDefinedName[13]":i8, "chUserDefinedName[14]":i8, "chUserDefinedName[15]":i8, "enDeviceType":i32, "nVendorId":u32, "nProductId":u32, "enUsbProtocol":i32, "chDeviceGUID[0]":i8, "chDeviceGUID[1]":i8, "chDeviceGUID[2]":i8, "chDeviceGUID[3]":i8, "chDeviceGUID[4]":i8, "chDeviceGUID[5]":i8, "chDeviceGUID[6]":i8, "chDeviceGUID[7]":i8, "chDeviceGUID[8]":i8, "chDeviceGUID[9]":i8, "chDeviceGUID[10]":i8, "chDeviceGUID[11]":i8, "chDeviceGUID[12]":i8, "chDeviceGUID[13]":i8, "chDeviceGUID[14]":i8, "chDeviceGUID[15]":i8, "chDeviceGUID[16]":i8, "chDeviceGUID[17]":i8, "chDeviceGUID[18]":i8, "chDeviceGUID[19]":i8, "chDeviceGUID[20]":i8, "chDeviceGUID[21]":i8, "chDeviceGUID[22]":i8, "chDeviceGUID[23]":i8, "chDeviceGUID[24]":i8, "chDeviceGUID[25]":i8, "chDeviceGUID[26]":i8, "chDeviceGUID[27]":i8, "chDeviceGUID[28]":i8, "chDeviceGUID[29]":i8, "chDeviceGUID[30]":i8, "chDeviceGUID[31]":i8, "chDeviceGUID[32]":i8, "chDeviceGUID[33]":i8, "chDeviceGUID[34]":i8, "chDeviceGUID[35]":i8, "chDeviceGUID[36]":i8, "chDeviceGUID[37]":i8, "chDeviceGUID[38]":i8, "chDeviceGUID[39]":i8, "chDeviceGUID[40]":i8, "chDeviceGUID[41]":i8, "chDeviceGUID[42]":i8, "chDeviceGUID[43]":i8, "chDeviceGUID[44]":i8, "chDeviceGUID[45]":i8, "chDeviceGUID[46]":i8, "chDeviceGUID[47]":i8, "chDeviceGUID[48]":i8, "chDeviceGUID[49]":i8, "chDeviceGUID[50]":i8, "chDeviceGUID[51]":i8, "chDeviceGUID[52]":i8, "chDeviceGUID[53]":i8, "chDeviceGUID[54]":i8, "chDeviceGUID[55]":i8, "chDeviceGUID[56]":i8, "chDeviceGUID[57]":i8, "chDeviceGUID[58]":i8, "chDeviceGUID[59]":i8, "chDeviceGUID[60]":i8, "chDeviceGUID[61]":i8, "chDeviceGUID[62]":i8, "chDeviceGUID[63]":i8, "nReserved[0]":u8, "nReserved[1]":u8, "nReserved[2]":u8, "nReserved[3]":u8, "nReserved[4]":u8, "nReserved[5]":u8, "nReserved[6]":u8, "nReserved[7]":u8, "nReserved[8]":u8, "nReserved[9]":u8, "nReserved[10]":u8, "nReserved[11]":u8, "nReserved[12]":u8, "nReserved[13]":u8, "nReserved[14]":u8, "nReserved[15]":u8}[]
  T13 = cluster{"enImageType":i32, "nWidth":u32, "nHeight":u32, "pData":u32, "nDataLen":u32, "nFrameNum":u32, "nTimeStamp":i64, "nReserved[0]":u8, "nReserved[1]":u8, "nReserved[2]":u8, "nReserved[3]":u8, "nReserved[4]":u8, "nReserved[5]":u8, "nReserved[6]":u8, "nReserved[7]":u8, "nReserved[8]":u8, "nReserved[9]":u8, "nReserved[10]":u8, "nReserved[11]":u8, "nReserved[12]":u8, "nReserved[13]":u8, "nReserved[14]":u8, "nReserved[15]":u8}[]
  T14 = typedef "imagedata.ctl" = cluster{"image type":i32, "image depth":i32, "image":u8[], "mask":u8[], "colors":u32[], "Rectangle":cluster{"left":i16, "top":i16, "right":i16, "bottom":i16}}
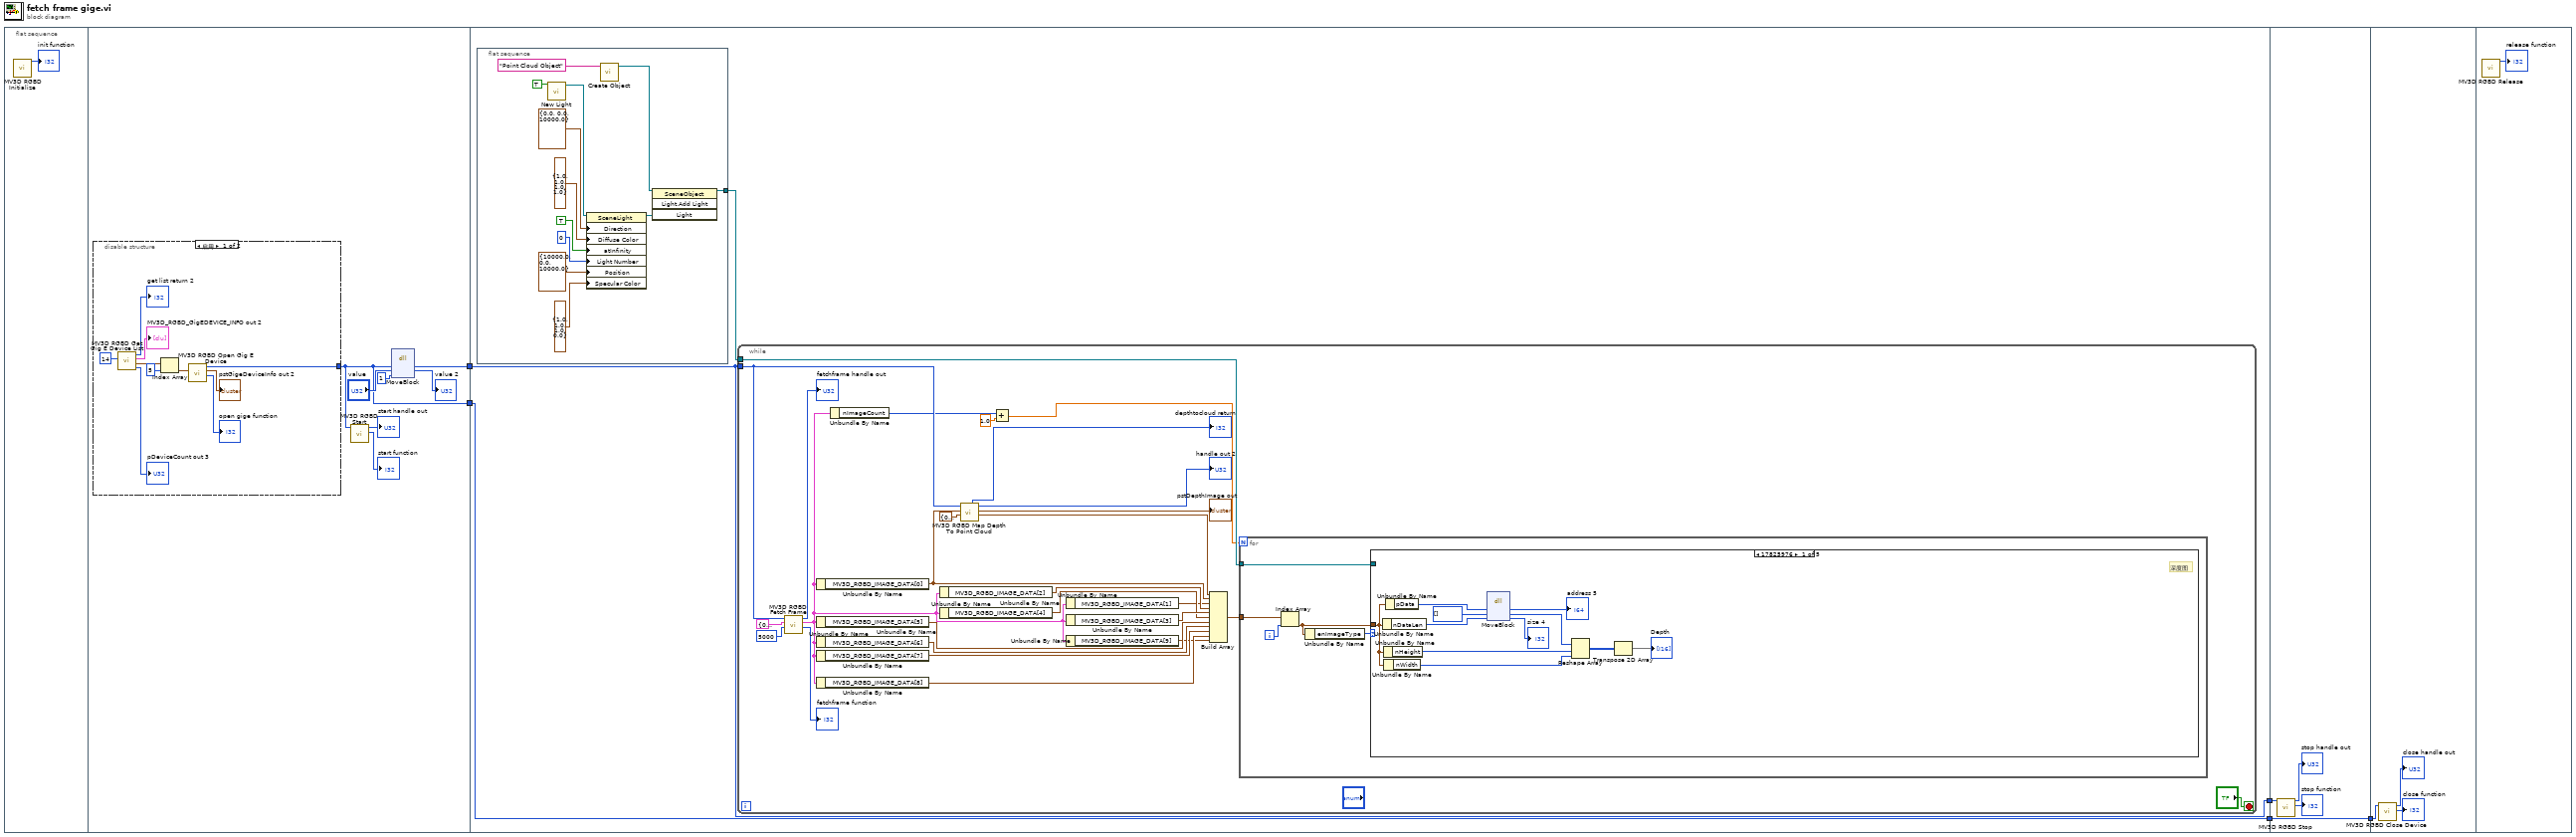
[diagram p0: block diagram]
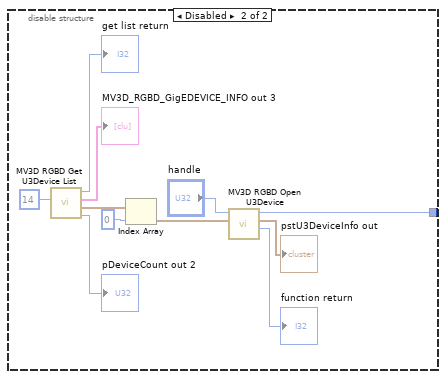
[diagram p2: hidden frame]
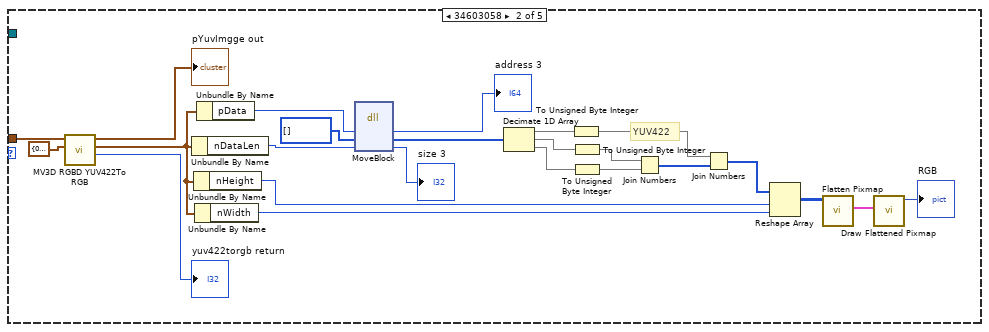
[diagram p3: hidden frame]
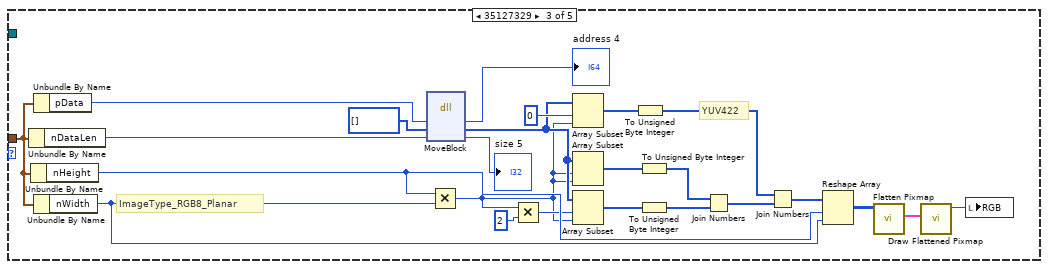
[diagram p4: hidden frame]
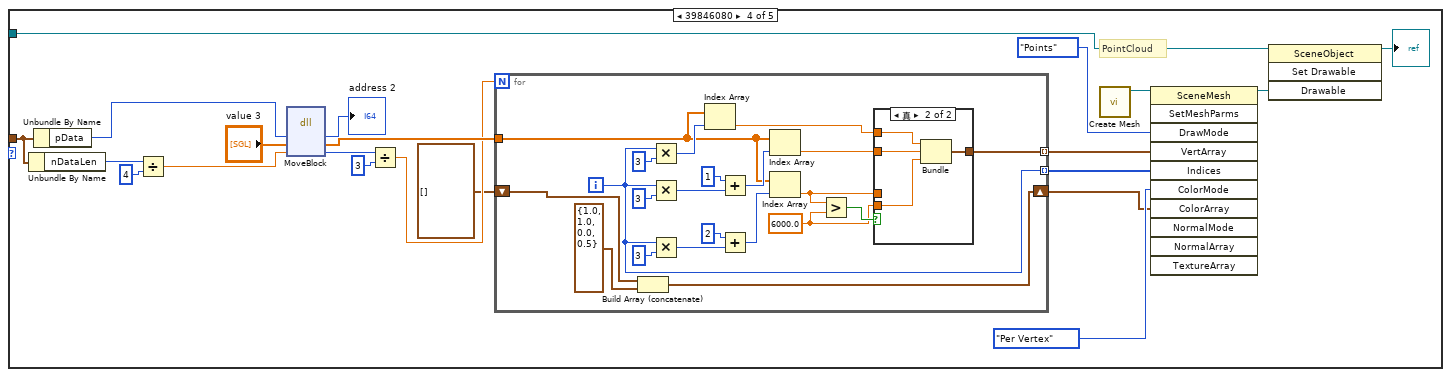
[diagram p5: hidden frame]
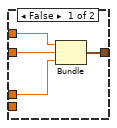
[diagram p6: hidden frame]
diagram:
  n1 = flat-sequence {
    tunnel: [w7] -> w3
    tunnel: [w9] -> w1
    tunnel: [w37] -> w4
    tunnel: w3 -> [w37]
    tunnel: [w35] -> w2
    tunnel: w1 -> [w35]
    tunnel: [w191] -> w5
    tunnel: w4 -> [w191]
    tunnel: w2 -> [w192]
    tunnel: w5 -> [w195]
    frame #0 {
      n2 = call <userlib>:"MV3D RGBD Initialize.vi"() -> ("function return"=→"init function":i32)  [unwired: 11 in]
    }
    frame #1 {
      n3 = disable-structure shown="启用" {
        disable-tunnel: [w14 w24] -> w7
        frame Enabled {
          n4 = call <userlib>:"MV3D RGBD Get Gig E Device List.vi"("nMaxDeviceCount"=u32 14) -> ("pDeviceCount out"=→"pDeviceCount out 3":u32, "MV3D_RGBD_GigEDEVICE_ByteINFO out"=w18:T11, "MV3D_RGBD_GigEDEVICE_INFO out"=→"MV3D_RGBD_GigEDEVICE_INFO out 2":T4, "function return"=→"get list return 2":i32)  [unwired: 7 in]
          n5 = Index Array(array=w18, index=5 ("设备索引")) -> (element=w17:T3)
          n6 = call <userlib>:"MV3D RGBD Open Gig E Device.vi"("pstGigeDeviceInfo 2"=w17) -> ("handle out"=w14:u32, "pstGigeDeviceInfo out"=→"pstGigeDeviceInfo out 2":T3, "function return"=→"open gige function":i32)  [unwired: 7 in]
        }
        frame Disabled {
          n7 = call <userlib>:"MV3D RGBD Get U3Device List.vi"("nMaxDeviceCount"=u32 14) -> ("pDeviceCount out"=→"pDeviceCount out 2":u32, "MV3D_RGBD_GigEDEVICE_ByteINFO out 2"=w29:T12, "MV3D_RGBD_GigEDEVICE_INFO out 2"=→"MV3D_RGBD_GigEDEVICE_INFO out 3":T2, "function return"=→"get list return":i32)  [unwired: 7 in]
          n8 = Index Array(array=w29, index=0 ("索引")) -> (element=w26:T1)
          n9 = call <userlib>:"MV3D RGBD Open U3Device.vi"("pstU3DeviceInfo"=w26, "handle"="handle") -> ("function return"=→"function return":i32, "pstU3DeviceInfo out"=→"pstU3DeviceInfo out":T1, "handle out"=w24:u32)  [unwired: 7 in]
        }
      }
      n10 = call <userlib>:"MV3D RGBD Start.vi"("handle"=w7) -> ("function return"=→"start function":i32, "handle out"=→"start handle out":u32)  [unwired: 9 in]
      n11 = dll-call lib="LabVIEW" fn="MoveBlock"("address"=w7, "value"="value", "size"=1) -> ("address"=w9:i64, "value"=→"value 2":u32)  [unwired: 5 in, 2 out]
    }
    frame #2 {
      n12 = flat-sequence {
        tunnel: [w47] -> w36
        frame #0 {
          n13 = call <vilib>:"New Light.vi"("At Infinity"=TRUE) -> ("New Light Refnum"=w44:refnum<vi>)  [unwired: 9 in, 1 out]
          n14 = property class="SceneLight"(reference=w44, "Direction"=T7 {"X"=0.0, "Y"=0.0, "Z"=10000.0} ("方向"), "Diffuse Color"=T6 {"Red"=1.0, "Green"=1.0, "Blue"=1.0, "Alpha"=1.0} ("散射光颜色"), "atInfinity"=TRUE ("位于无穷远处"), "Light Number"=0 ("光源编号"), "Position"=T7 {"X"=10000.0, "Y"=0.0, "Z"=10000.0} ("位置"), "Specular Color"=T6 {"Red"=1.0, "Green"=1.0, "Blue"=1.0, "Alpha"=0.0} ("反光颜色")) -> (reference out=w46:refnum<vi>)  [unwired: 1 in, 1 out]
          n15 = call-poly <vilib>:"Create Object.vi"("Name"="Point Cloud Object") -> ("Scene:New Object"=w48:refnum<vi>)  [unwired: 9 in, 1 out]
          n16 = invoke class="SceneObject" method="Light.Add Light"(reference=w48, "Light"=w46) -> (reference out=w47:refnum<vi>)  [unwired: 2 in, 3 out]
        }
      }
      n17 = while {
        tunnel: w35 -> [w68]
        tunnel: w36 -> [w54]
        stop <- "?" stop-if-true
        n18 = call <userlib>:"MV3D RGBD Fetch Frame.vi"("nTimeOut"=u32 5000, "pstFrameData"=T8 {"nImageCount"=0, "MV3D_RGBD_IMAGE_DATA[0]"={"enImageType"=0, "nWidth"=0, "nHeight"=0, "pData"=0, "nDataLen"=0, "nFrameNum"=0, "nTimeStamp"=0, "nReserved[0]"=0, "nReserved[1]"=0, "nReserved[2]"=0, "nReserved[3]"=0, "nReserved[4]"=0, "nReserved[5]"=0, "nReserved[6]"=0, "nReserved[7]"=0, "nReserved[8]"=0, "nReserved[9]"=0, "nReserved[10]"=0, "nReserved[11]"=0, "nReserved[12]"=0, "nReserved[13]"=0, "nReserved[14]"=0, "nReserved[15]"=0}, "MV3D_RGBD_IMAGE_DATA[1]"={"enImageType"=0, "nWidth"=0, "nHeight"=0, "pData"=0, "nDataLen"=0, "nFrameNum"=0, "nTimeStamp"=0, "nReserved[0]"=0, "nReserved[1]"=0, "nReserved[2]"=0, "nReserved[3]"=0, "nReserved[4]"=0, "nReserved[5]"=0, "nReserved[6]"=0, "nReserved[7]"=0, "nReserved[8]"=0, "nReserved[9]"=0, "nReserved[10]"=0, "nReserved[11]"=0, "nReserved[12]"=0, "nReserved[13]"=0, "nReserved[14]"=0, "nReserved[15]"=0}, "MV3D_RGBD_IMAGE_DATA[2]"={"enImageType"=0, "nWidth"=0, "nHeight"=0, "pData"=0, "nDataLen"=0, "nFrameNum"=0, "nTimeStamp"=0, "nReserved[0]"=0, "nReserved[1]"=0, "nReserved[2]"=0, "nReserved[3]"=0, "nReserved[4]"=0, "nReserved[5]"=0, "nReserved[6]"=0, "nReserved[7]"=0, "nReserved[8]"=0, "nReserved[9]"=0, "nReserved[10]"=0, "nReserved[11]"=0, "nReserved[12]"=0, "nReserved[13]"=0, "nReserved[14]"=0, "nReserved[15]"=0}, "MV3D_RGBD_IMAGE_DATA[3]"={"enImageType"=0, "nWidth"=0, "nHeight"=0, "pData"=0, "nDataLen"=0, "nFrameNum"=0, "nTimeStamp"=0, "nReserved[0]"=0, "nReserved[1]"=0, "nReserved[2]"=0, "nReserved[3]"=0, "nReserved[4]"=0, "nReserved[5]"=0, "nReserved[6]"=0, "nReserved[7]"=0, "nReserved[8]"=0, "nReserved[9]"=0, "nReserved[10]"=0, "nReserved[11]"=0, "nReserved[12]"=0, "nReserved[13]"=0, "nReserved[14]"=0, "nReserved[15]"=0}, "MV3D_RGBD_IMAGE_DATA[4]"={"enImageType"=0, "nWidth"=0, "nHeight"=0, "pData"=0, "nDataLen"=0, "nFrameNum"=0, "nTimeStamp"=0, "nReserved[0]"=0, "nReserved[1]"=0, "nReserved[2]"=0, "nReserved[3]"=0, "nReserved[4]"=0, "nReserved[5]"=0, "nReserved[6]"=0, "nReserved[7]"=0, "nReserved[8]"=0, "nReserved[9]"=0, "nReserved[10]"=0, "nReserved[11]"=0, "nReserved[12]"=0, "nReserved[13]"=0, "nReserved[14]"=0, "nReserved[15]"=0}, "MV3D_RGBD_IMAGE_DATA[5]"={"enImageType"=0, "nWidth"=0, "nHeight"=0, "pData"=0, "nDataLen"=0, "nFrameNum"=0, "nTimeStamp"=0, "nReserved[0]"=0, "nReserved[1]"=0, "nReserved[2]"=0, "nReserved[3]"=0, "nReserved[4]"=0, "nReserved[5]"=0, "nReserved[6]"=0, "nReserved[7]"=0, "nReserved[8]"=0, "nReserved[9]"=0, "nReserved[10]"=0, "nReserved[11]"=0, "nReserved[12]"=0, "nReserved[13]"=0, "nReserved[14]"=0, "nReserved[15]"=0}, "MV3D_RGBD_IMAGE_DATA[6]"={"enImageType"=0, "nWidth"=0, "nHeight"=0, "pData"=0, "nDataLen"=0, "nFrameNum"=0, "nTimeStamp"=0, "nReserved[0]"=0, "nReserved[1]"=0, "nReserved[2]"=0, "nReserved[3]"=0, "nReserved[4]"=0, "nReserved[5]"=0, "nReserved[6]"=0, "nReserved[7]"=0, "nReserved[8]"=0, "nReserved[9]"=0, "nReserved[10]"=0, "nReserved[11]"=0, "nReserved[12]"=0, "nReserved[13]"=0, "nReserved[14]"=0, "nReserved[15]"=0}, "MV3D_RGBD_IMAGE_DATA[7]"={"enImageType"=0, "nWidth"=0, "nHeight"=0, "pData"=0, "nDataLen"=0, "nFrameNum"=0, "nTimeStamp"=0, "nReserved[0]"=0, "nReserved[1]"=0, "nReserved[2]"=0, "nReserved[3]"=0, "nReserved[4]"=0, "nReserved[5]"=0, "nReserved[6]"=0, "nReserved[7]"=0, "nReserved[8]"=0, "nReserved[9]"=0, "nReserved[10]"=0, "nReserved[11]"=0, "nReserved[12]"=0, "nReserved[13]"=0, "nReserved[14]"=0, "nReserved[15]"=0}, "MV3D_RGBD_IMAGE_DATA[8]"={"enImageType"=0, "nWidth"=0, "nHeight"=0, "pData"=0, "nDataLen"=0, "nFrameNum"=0, "nTimeStamp"=0, "nReserved[0]"=0, "nReserved[1]"=0, "nReserved[2]"=0, "nReserved[3]"=0, "nReserved[4]"=0, "nReserved[5]"=0, "nReserved[6]"=0, "nReserved[7]"=0, "nReserved[8]"=0, "nReserved[9]"=0, "nReserved[10]"=0, "nReserved[11]"=0, "nReserved[12]"=0, "nReserved[13]"=0, "nReserved[14]"=0, "nReserved[15]"=0}, "MV3D_RGBD_IMAGE_DATA[9]"={"enImageType"=0, "nWidth"=0, "nHeight"=0, "pData"=0, "nDataLen"=0, "nFrameNum"=0, "nTimeStamp"=0, "nReserved[0]"=0, "nReserved[1]"=0, "nReserved[2]"=0, "nReserved[3]"=0, "nReserved[4]"=0, "nReserved[5]"=0, "nReserved[6]"=0, "nReserved[7]"=0, "nReserved[8]"=0, "nReserved[9]"=0, "nReserved[10]"=0, "nReserved[11]"=0, "nReserved[12]"=0, "nReserved[13]"=0, "nReserved[14]"=0, "nReserved[15]"=0}, "nReserved[0]"=0, "nReserved[1]"=0, "nReserved[2]"=0, "nReserved[3]"=0, "nReserved[4]"=0, "nReserved[5]"=0, "nReserved[6]"=0, "nReserved[7]"=0, "nReserved[8]"=0, "nReserved[9]"=0, "nReserved[10]"=0, "nReserved[11]"=0, "nReserved[12]"=0, "nReserved[13]"=0, "nReserved[14]"=0, "nReserved[15]"=0}, "handle"=w68) -> ("function return"=→"fetchframe function":i32, "pstFrameData out"=w56:T8, "handle out"=→"fetchframe handle out":u32)  [unwired: 6 in]
        n19 = Unbundle By Name(w56) -> ("MV3D_RGBD_IMAGE_DATA[0]"=w66:T5)
        n20 = Unbundle By Name(w56) -> ("MV3D_RGBD_IMAGE_DATA[5]"=w62:T5)
        n21 = Unbundle By Name(w56) -> ("MV3D_RGBD_IMAGE_DATA[6]"=w61:T5)
        n22 = Unbundle By Name(w56) -> ("MV3D_RGBD_IMAGE_DATA[7]"=w60:T5)
        n23 = Unbundle By Name(w56) -> ("MV3D_RGBD_IMAGE_DATA[8]"=w59:T5)
        n24 = Unbundle By Name(w56) -> ("nImageCount"=w51:u64)
        n25 = Unbundle By Name(w56) -> ("MV3D_RGBD_IMAGE_DATA[2]"=w65:T5)
        n26 = Unbundle By Name(w56) -> ("MV3D_RGBD_IMAGE_DATA[4]"=w63:T5)
        n27 = call <userlib>:"MV3D RGBD Map Depth To Point Cloud.vi"("pstPointCloudImage"=T5 {"enImageType"=0, "nWidth"=0, "nHeight"=0, "pData"=0, "nDataLen"=0, "nFrameNum"=0, "nTimeStamp"=0, "nReserved[0]"=0, "nReserved[1]"=0, "nReserved[2]"=0, "nReserved[3]"=0, "nReserved[4]"=0, "nReserved[5]"=0, "nReserved[6]"=0, "nReserved[7]"=0, "nReserved[8]"=0, "nReserved[9]"=0, "nReserved[10]"=0, "nReserved[11]"=0, "nReserved[12]"=0, "nReserved[13]"=0, "nReserved[14]"=0, "nReserved[15]"=0}, "pstDepthImage"=w66, "handle"=w68) -> ("pstPointCloudImage out"=w53:T5, "pstDepthImage out"=→"pstDepthImage out":T5, "handle out"=→"handle out 2":u32, "function return"=→"depthtocloud return":i32)  [unwired: 5 in]
        n28 = Add(x=w51, y=1.0) -> (x+y=w50:dbl)
        n29 = Unbundle By Name(w56) -> ("MV3D_RGBD_IMAGE_DATA[1]"=w58:T5)
        n30 = Unbundle By Name(w56) -> ("MV3D_RGBD_IMAGE_DATA[3]"=w64:T5)
        n31 = Unbundle By Name(w56) -> ("MV3D_RGBD_IMAGE_DATA[9]"=w57:T5)
        n32 = Build Array(w53, w66, w58, w65, w64, w63, w62, w61, w60, w59, w57) -> (w55:T13)
        n33 = for {
          N: w50 -> [_]
          tunnel: w55 -> [w80]
          tunnel: w54 -> [w78]
          i -> [w81]
          n34 = Index Array(array=w80, index=w81) -> (element=w77:T5)
          n35 = Unbundle By Name(w77) -> ("enImageType"=w79:i32)
          n36 = case shown="17825976" w79 {
            tunnel: w77 -> [w86 w94 w128 w151 _]
            tunnel: w78 -> [_ _ _ w147 _]
            frame 17825976 {
              # "深度图"
              n37 = Unbundle By Name(w86) -> ("nDataLen"=w82:u32)
              n38 = Unbundle By Name(w86) -> ("nHeight"=w84:u32)
              n39 = Unbundle By Name(w86) -> ("nWidth"=w83:u32)
              n40 = Unbundle By Name(w86) -> ("pData"=w85:u32)
              n41 = dll-call lib="LabVIEW" fn="MoveBlock"("address"=w85, "value"=i16[] [] ("value 6"), "size"=w82) -> ("address"=→"address 5":i64, "value"=w90:i16[], "size"=→"size 4":i32)  [unwired: 4 in, 2 out]
              n42 = Reshape Array(w90, w84, w83) -> (w91:i16[][])
              n43 = Transpose 2D Array(2D array=w91) -> (transposed array=→"Depth":i16[][])
            }
            frame 34603058 {
              # "YUV422"
              n44 = call <userlib>:"MV3D RGBD YUV422To RGB.vi"("pRgbImage"=T5 {"enImageType"=0, "nWidth"=0, "nHeight"=0, "pData"=0, "nDataLen"=0, "nFrameNum"=0, "nTimeStamp"=0, "nReserved[0]"=0, "nReserved[1]"=0, "nReserved[2]"=0, "nReserved[3]"=0, "nReserved[4]"=0, "nReserved[5]"=0, "nReserved[6]"=0, "nReserved[7]"=0, "nReserved[8]"=0, "nReserved[9]"=0, "nReserved[10]"=0, "nReserved[11]"=0, "nReserved[12]"=0, "nReserved[13]"=0, "nReserved[14]"=0, "nReserved[15]"=0}, "pYuvImgge"=w94) -> ("function return"=→"yuv422torgb return":i32, "pRgbImage out"=w95:T5, "pYuvImgge out"=→"pYuvImgge out":T5)  [unwired: 7 in]
              n45 = Unbundle By Name(w95) -> ("nDataLen"=w100:u32)
              n46 = Unbundle By Name(w95) -> ("nHeight"=w109:u32)
              n47 = Unbundle By Name(w95) -> ("nWidth"=w108:u32)
              n48 = Unbundle By Name(w95) -> ("pData"=w99:u32)
              n49 = dll-call lib="LabVIEW" fn="MoveBlock"("address"=w99, "value"=i16[] [] ("value 5"), "size"=w100) -> ("address"=→"address 3":i64, "value"=w101:u8[], "size"=→"size 3":i32)  [unwired: 4 in, 2 out]
              n50 = Decimate 1D Array(w101) -> (w102:u8[], w103:u8[], w104:u8[])
              n51 = To Unsigned Byte Integer(number=w102) -> (unsigned 8bit integer=w112:u8[])
              n52 = To Unsigned Byte Integer(number=w103) -> (unsigned 8bit integer=w110:u8[])
              n53 = To Unsigned Byte Integer(number=w104) -> (unsigned 8bit integer=w113:u8[])
              n54 = Join Numbers(hi=w110, lo=w113) -> ((hi.lo)=w111:u16[])
              n55 = Join Numbers(hi=w112, lo=w111) -> ((hi.lo)=w105:u32[])
              n56 = Reshape Array(w105, w109, w108) -> (w106:u32[][])
              n57 = call <vilib>:"Flatten Pixmap.vi"("24-bit pixmap"=w106) -> ("image data"=w107:T14)  [unwired: 10 in]
              n58 = call <vilib>:"Draw Flattened Pixmap.vi"("image data"=w107) -> ("new picture"=→"RGB":picture)  [unwired: 8 in]
            }
            frame 35127329 {
              # "YUV422"
              # "ImageType_RGB8_Planar"
              n59 = Unbundle By Name(w128) -> ("nDataLen"=w133:u32)
              n60 = Unbundle By Name(w128) -> ("nHeight"=w122:u32)
              n61 = Unbundle By Name(w128) -> ("pData"=w132:u32)
              n62 = Unbundle By Name(w128) -> ("nWidth"=w121:u32)
              n63 = dll-call lib="LabVIEW" fn="MoveBlock"("address"=w132, "value"=i16[] [] ("value 5"), "size"=w133) -> ("address"=→"address 4":i64, "value"=w123:u8[], "size"=→"size 5":i32)  [unwired: 4 in, 2 out]
              n64 = Multiply(x=w122, y=w121) -> (x*y=w118:u32)
              n65 = Multiply(x=w118, y=u32 2) -> (x*y=w119:u32)
              n66 = Array Subset(array=w123, index=0 ("索引"), length=w118) -> (w126:u8[])
              n67 = Array Subset(array=w123, index=w118, length=w118) -> (w125:u8[])
              n68 = Array Subset(array=w123, index=w119, length=w118) -> (w124:u8[])
              n69 = To Unsigned Byte Integer(number=w126) -> (unsigned 8bit integer=w139:u8[])
              n70 = To Unsigned Byte Integer(number=w125) -> (unsigned 8bit integer=w137:u8[])
              n71 = To Unsigned Byte Integer(number=w124) -> (unsigned 8bit integer=w140:u8[])
              n72 = Join Numbers(hi=w137, lo=w140) -> ((hi.lo)=w138:u16[])
              n73 = Join Numbers(hi=w139, lo=w138) -> ((hi.lo)=w134:u32[])
              n74 = Reshape Array(w134, w122, w121) -> (w135:u32[][])
              n75 = call <vilib>:"Flatten Pixmap.vi"("24-bit pixmap"=w135) -> ("image data"=w136:T14)  [unwired: 10 in]
              n76 = call <vilib>:"Draw Flattened Pixmap.vi"("image data"=w136) -> ("new picture"=w117:picture)  [unwired: 8 in]
              n77 = local write "RGB"(w117) -> ()
            }
            frame 39846080 {
              # "PointCloud"
              n78 = Unbundle By Name(w151) -> ("nDataLen"=w158:u32)
              n79 = Unbundle By Name(w151) -> ("pData"=w159:u32)
              n80 = Divide(x=w158, y=u32 4) -> (x/y=w156:dbl)
              n81 = dll-call lib="LabVIEW" fn="MoveBlock"("address"=w159, "value"="value 3", "size"=w156) -> ("address"=→"address 2":i64, "value"=w150:sgl[], "size"=w145:i32)  [unwired: 4 in, 2 out]
              n82 = Divide(x=w145, y=3) -> (x/y=w144:dbl)
              n83 = for {
                N: w144 -> [_]
                tunnel: [w163] -> w149 mode=indexing
                tunnel: [w172] -> w148 mode=indexing
                tunnel: w150 -> [w171]
                shift-right: [w168] -> w141
                shift-left: T6[] [] ("颜色数组") -> [w169]
                i -> [w172]
                w162 = sgl 6000.0 ("y")
                n84 = Build Array (concatenate)(w169, T6 {"Red"=1.0, "Green"=1.0, "Blue"=0.0, "Alpha"=0.5} ("Color")) -> (w168:T6[])
                n85 = Multiply(x=w172, y=3) -> (x*y=w181:i32)
                n86 = Multiply(x=w172, y=3) -> (x*y=w179:i32)
                n87 = Multiply(x=w172, y=3) -> (x*y=w175:i32)
                n88 = Index Array(array=w171, index=w181) -> (element=w166:sgl)
                n89 = Add(x=1, y=w179) -> (x+y=w177:i32)
                n90 = Add(x=2, y=w175) -> (x+y=w173:i32)
                n91 = Index Array(array=w171, index=w177) -> (element=w165:sgl)
                n92 = Index Array(array=w171, index=w173) -> (element=w164:sgl)
                n93 = Greater?(x=w164, y=w162) -> (0:w167:bool)
                n94 = case shown="真" w167 {
                  tunnel: w166 -> [w186 w190]
                  tunnel: w165 -> [w185 w189]
                  tunnel: w164 -> [w184 _]
                  tunnel: [w183 w187] -> w163
                  tunnel: w162 -> [_ w188]
                  frame False {
                    n95 = Bundle(w186, w185, w184) -> (w183:cluster{sgl, sgl, sgl})  [unwired: 1 in]
                  }
                  frame True {
                    n96 = Bundle(w190, w189, "y"=w188) -> (w187:cluster{sgl, sgl, "y":sgl})  [unwired: 1 in]
                  }
                }
              }
              n97 = call <vilib>:"Create Mesh.vi"() -> ("New Mesh Refnum"=w155:refnum<vi>)  [unwired: 10 in, 1 out]
              n98 = invoke class="SceneMesh" method="SetMeshParms"(reference=w155, "DrawMode"=T10."Points" ("绘图模式"), "VertArray"=w149, "Indices"=w148, "ColorMode"=T9."Per Vertex" ("颜色绑定模式"), "ColorArray"=w141) -> (reference out=w153:refnum<vi>)  [unwired: 5 in, 10 out]
              n99 = invoke class="SceneObject" method="Set Drawable"(reference=w147, "Drawable"=w153) -> (reference out=→"?":refnum<vi>)  [unwired: 2 in, 3 out]
            }
            frame 0, Default {
            }
          }
        }
      }
    }
    frame #3 {
      n100 = call <userlib>:"MV3D RGBD Stop.vi"("handle"=w192) -> ("function return"=→"stop function":i32, "handle out"=→"stop handle out":u32)  [unwired: 9 in]
    }
    frame #4 {
      n101 = call <userlib>:"MV3D RGBD Close Device.vi"("handle"=w195) -> ("function return"=→"close function":i32, "handle out"=→"close handle out":u32)  [unwired: 9 in]
    }
    frame #5 {
      n102 = call <userlib>:"MV3D RGBD Release.vi"() -> ("function return"=→"release function":i32)  [unwired: 11 in]
    }
  }
